vi "RichToFlatgrpc_reflection_v1alpha_ServerReflectionResponse.vi"(5 "OutputClusterType":T1, 11 "InputCluster":T9) -> (3 "OutputCluster":T1)   [LabVIEW 2025, in "reflection_server.lvlib"]
uses:
  reflection_server.lvlib
  grpc_reflection_v1alpha_ServerReflectionResponse.ctl
  grpc_reflection_v1alpha_ServerReflectionRequest_message_request/grpc_reflection_v1alpha_ServerReflectionRequest_message_request.lvclass
  grpc_reflection_v1alpha_ServerReflectionResponse_message_response/grpc_reflection_v1alpha_ServerReflectionResponse_message_response.lvclass
  grpc_reflection_v1alpha_ServerReflectionRequest.ctl
  grpc_reflection_v1alpha_ServerReflectionResponse_Flat.ctl
  grpc_reflection_v1alpha_ServerReflectionRequest_Flat.ctl
  grpc_reflection_v1alpha_ExtensionRequest_Flat.ctl
  grpc_reflection_v1alpha_FileDescriptorResponse_Flat.ctl
  grpc_reflection_v1alpha_ExtensionNumberResponse_Flat.ctl
  grpc_reflection_v1alpha_ListServiceResponse_Flat.ctl
  grpc_reflection_v1alpha_ServiceResponse_Flat.ctl
  grpc_reflection_v1alpha_ErrorResponse_Flat.ctl
  grpc_reflection_v1alpha_ServerReflectionRequest_message_request/grpc_reflection_v1alpha_ServerReflectionRequest_message_request.lvclass/grpc_reflection_v1alpha_ServerReflectionRequest_message_request.ctl
  grpc_reflection_v1alpha_ServerReflectionResponse_message_response/grpc_reflection_v1alpha_ServerReflectionResponse_message_response.lvclass/grpc_reflection_v1alpha_ServerReflectionResponse_message_response.ctl
  grpc_reflection_v1alpha_ServerReflectionRequest_message_request/Getfile_by_filename.vi
  grpc_reflection_v1alpha_ServerReflectionRequest_message_request/Getfile_containing_symbol.vi
  grpc_reflection_v1alpha_ServerReflectionRequest_message_request/Getfile_containing_extension.vi
  RichToFlatgrpc_reflection_v1alpha_ExtensionRequest.vi
  grpc_reflection_v1alpha_ServerReflectionRequest_message_request/Getall_extension_numbers_of_type.vi
  grpc_reflection_v1alpha_ServerReflectionRequest_message_request/Getlist_services.vi
  RichToFlatgrpc_reflection_v1alpha_ServiceResponse.vi
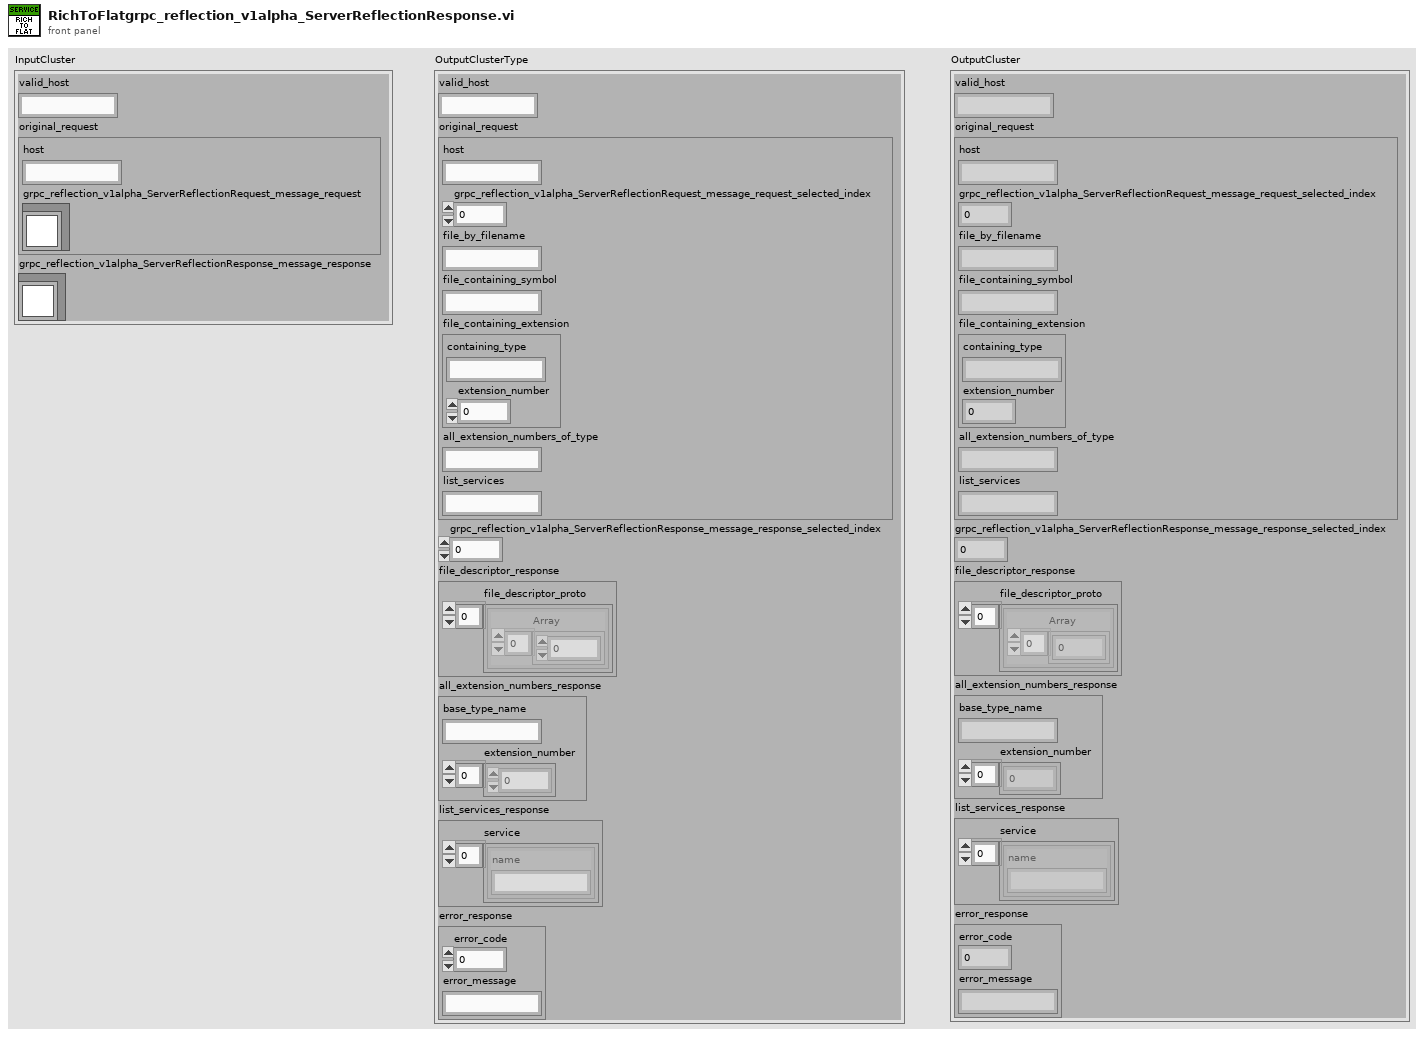
[diagram p1: front panel]
types:
  T1 = typedef "reflection_server.lvlib/grpc_reflection_v1alpha_ServerReflectionResponse_Flat.ctl" = cluster{"valid_host":string, "original_request":T2, "grpc_reflection_v1alpha_ServerReflectionResponse_message_response_selected_index":i32, "file_descriptor_response":T4, "all_extension_numbers_response":T5, "list_services_response":T6, "error_response":T8}
  T2 = typedef "reflection_server.lvlib/grpc_reflection_v1alpha_ServerReflectionRequest_Flat.ctl" = cluster{"host":string, "grpc_reflection_v1alpha_ServerReflectionRequest_message_request_selected_index":i32, "file_by_filename":string, "file_containing_symbol":string, "file_containing_extension":T3, "all_extension_numbers_of_type":string, "list_services":string}
  T3 = typedef "reflection_server.lvlib/grpc_reflection_v1alpha_ExtensionRequest_Flat.ctl" = cluster{"containing_type":string, "extension_number":i32}
  T4 = typedef "reflection_server.lvlib/grpc_reflection_v1alpha_FileDescriptorResponse_Flat.ctl" = cluster{"file_descriptor_proto":cluster{"Array":u8[]}[]}
  T5 = typedef "reflection_server.lvlib/grpc_reflection_v1alpha_ExtensionNumberResponse_Flat.ctl" = cluster{"base_type_name":string, "extension_number":i32[]}
  T6 = typedef "reflection_server.lvlib/grpc_reflection_v1alpha_ListServiceResponse_Flat.ctl" = cluster{"service":T7[]}
  T7 = typedef "reflection_server.lvlib/grpc_reflection_v1alpha_ServiceResponse_Flat.ctl" = cluster{"name":string}
  T8 = typedef "reflection_server.lvlib/grpc_reflection_v1alpha_ErrorResponse_Flat.ctl" = cluster{"error_code":i32, "error_message":string}
  T9 = typedef "reflection_server.lvlib/grpc_reflection_v1alpha_ServerReflectionResponse.ctl" = cluster{"valid_host":string, "original_request":T10, "grpc_reflection_v1alpha_ServerReflectionResponse_message_response":refnum<class "grpc_reflection_v1alpha_ServerReflectionResponse_message_response.lvclass">}
  T10 = typedef "reflection_server.lvlib/grpc_reflection_v1alpha_ServerReflectionRequest.ctl" = cluster{"host":string, "grpc_reflection_v1alpha_ServerReflectionRequest_message_request":refnum<class "grpc_reflection_v1alpha_ServerReflectionRequest_message_request.lvclass">}
  T11 = typedef "reflection_server.lvlib/grpc_reflection_v1alpha_FileDescriptorResponse.ctl" = cluster{"file_descriptor_proto":cluster{"Array":u8[]}[]}
  T12 = typedef "reflection_server.lvlib/grpc_reflection_v1alpha_ExtensionNumberResponse.ctl" = cluster{"base_type_name":string, "extension_number":i32[]}
  T13 = typedef "reflection_server.lvlib/grpc_reflection_v1alpha_ListServiceResponse.ctl" = cluster{"service":T14[]}
  T14 = typedef "reflection_server.lvlib/grpc_reflection_v1alpha_ServiceResponse.ctl" = cluster{"name":string}
  T15 = typedef "reflection_server.lvlib/grpc_reflection_v1alpha_ErrorResponse.ctl" = cluster{"error_code":i32, "error_message":string}
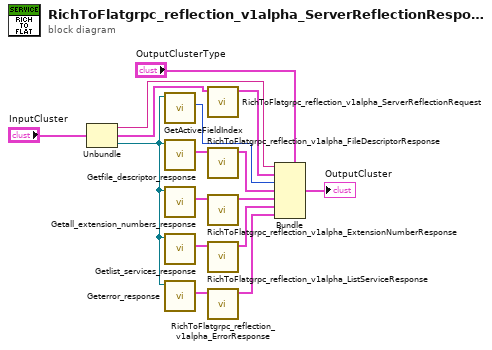
[diagram p0: block diagram]
diagram:
  n1 = Unbundle "Unbundle"("InputCluster") -> ("valid_host"=w13:string, "original_request"=w12:T10, "grpc_reflection_v1alpha_ServerReflectionResponse_message_response"=w10:refnum<class "grpc_reflection_v1alpha_ServerReflectionResponse_message_response.lvclass">)
  n2 = call "GetActiveFieldIndex.vi"("OneOfTemplate in"=w10) -> ("Active Field Index"=w9:i32)  [unwired: 8 in, 2 out]
  n3 = call "Getfile_descriptor_response.vi"("OneOfTemplate in"=w10) -> ("Get_Val"=w8:T11)  [unwired: 8 in, 2 out]
  n4 = call "Getall_extension_numbers_response.vi"("OneOfTemplate in"=w10) -> ("Get_Val"=w6:T12)  [unwired: 8 in, 2 out]
  n5 = call "Getlist_services_response.vi"("OneOfTemplate in"=w10) -> ("Get_Val"=w4:T13)  [unwired: 8 in, 2 out]
  n6 = call "Geterror_response.vi"("OneOfTemplate in"=w10) -> ("Get_Val"=w2:T15)  [unwired: 8 in, 2 out]
  n7 = call "RichToFlatgrpc_reflection_v1alpha_ServerReflectionRequest.vi"("InputCluster"=w12) -> ("OutputCluster"=w11:T2)  [unwired: 10 in]
  n8 = call "RichToFlatgrpc_reflection_v1alpha_FileDescriptorResponse.vi"("InputCluster"=w8) -> ("OutputCluster"=w7:T4)  [unwired: 10 in]
  n9 = call "RichToFlatgrpc_reflection_v1alpha_ExtensionNumberResponse.vi"("InputCluster"=w6) -> ("OutputCluster"=w5:T5)  [unwired: 10 in]
  n10 = call "RichToFlatgrpc_reflection_v1alpha_ListServiceResponse.vi"("InputCluster"=w4) -> ("OutputCluster"=w3:T6)  [unwired: 10 in]
  n11 = call "RichToFlatgrpc_reflection_v1alpha_ErrorResponse.vi"("InputCluster"=w2) -> ("OutputCluster"=w1:T8)  [unwired: 10 in]
  n12 = Bundle "Bundle"(cluster="OutputClusterType", "valid_host"=w13, "original_request"=w11, "grpc_reflection_v1alpha_ServerReflectionResponse_message_response_selected_index"=w9, "file_descriptor_response"=w7, "all_extension_numbers_response"=w5, "list_services_response"=w3, "error_response"=w1) -> (→"OutputCluster":T1)
